vi "DAQ_DC-RMS Current Meas Configure and Measure.vi"(0 "DAQmx Task In":refnum<k21>, 2 "Execution Settings":T2, 5 "Range and Terminal Settings":T7={"Global Settings"={"Min Range (A)"=-0.01, "Max Range (A)"=0.01, "Terminal Configuration"=10083, "Shunt Resistor (Ohm)"=0.001}, "Specific Channel Settings"=[]} {"Specific Channel Settings"."Shunt Resistor (ohms)" format="%.2p"; "Specific Channel Settings"."Terminal Configuration" items=["RSE"=10083, "NRSE"=10078, "Differential"=10106]; "Specific Channel Settings"."Max Range" format="%.2p"; "Specific Channel Settings"."Min Range" format="%.2p"; "Global Settings"."Shunt Resistor (Ohm)" format="%.2p"; "Global Settings"."Terminal Configuration" items=["RSE"=10083, "NRSE"=10078, "Differential"=10106]; "Global Settings"."Max Range (A)" format="%.2p"; "Global Settings"."Min Range (A)" format="%.2p"}, 7 "Timing & Trigger Settings":T4={"Timing Settings"={"Sample Clock Source"="OnboardClock", "Sample Rate (Hz)"=10000.0, "Number of Samples"=1000, "Sample Timing Engine"=enum."Auto"}, "Trigger Settings"={"Trigger Type"=enum."No Trigger", "Digital Start Trigger Source"="", "Digital Start Trigger Edge"=10280}} {"Trigger Settings"."Digital Start Trigger Edge" items=["Rising"=10280, "Falling"=10171]; "Timing Settings"."Sample Rate (Hz)" format="%.2p"}, 11 "error in":errorcluster) -> (4 "DAQmx Task Out":refnum<k21>, 6 "DC and RMS Current Measurements":T1 {"RMS Current (A)" format="%#.2p"; "Average DC Current (A)" format="%#.2p"}, 8 "Current Waveforms":waveform(dbl)[](graph), 10 "Acquisition Time (s)":dbl format="%.2p", 15 "error out":errorcluster)   [LabVIEW 2021, in "DAQ_DC-RMS Current Measurement.lvlib"]
doc: "Configure, initiate and fetch DC-RMS Current measurements from the channels configured."
uses:
  DAQ_DC-RMS Current Measurement.lvlib
  Typedefs/Range and Terminal Settings.ctl
  Typedefs/Specific Channel Settings.ctl
  Typedefs/Timing & Trigger Settings.ctl
  Typedefs/Timing Settings.ctl
  Typedefs/Trigger Settings.ctl
  Typedefs/Execution Settings.ctl
  Common/Typedefs/Execution Options - Measure.ctl
  Typedefs/DC and RMS Current Measurements.ctl
  <vilib>/DAQmx/read.llb/DAQmx Read (Analog 1D Wfm NChan NSamp).vi
  <vilib>/DAQmx/configure/timing.llb/DAQmx Timing (Sample Clock).vi
  <vilib>/DAQmx/configure/trigger.llb/DAQmx Start Trigger (Digital Edge).vi
  <vilib>/DAQmx/miscellaneous.llb/DAQmx Fill In Error Info.vi
  <resource>/objmgr/daqmx.rc
panel:
  # "Inputs"
  # "Outputs"
  # "Min. Range(A)"
  # "Max. Range(A)"
  # "Terminal Configuration"
  # "Shunt\nResistor(Ohm)"
  # "Physical Channel Name"
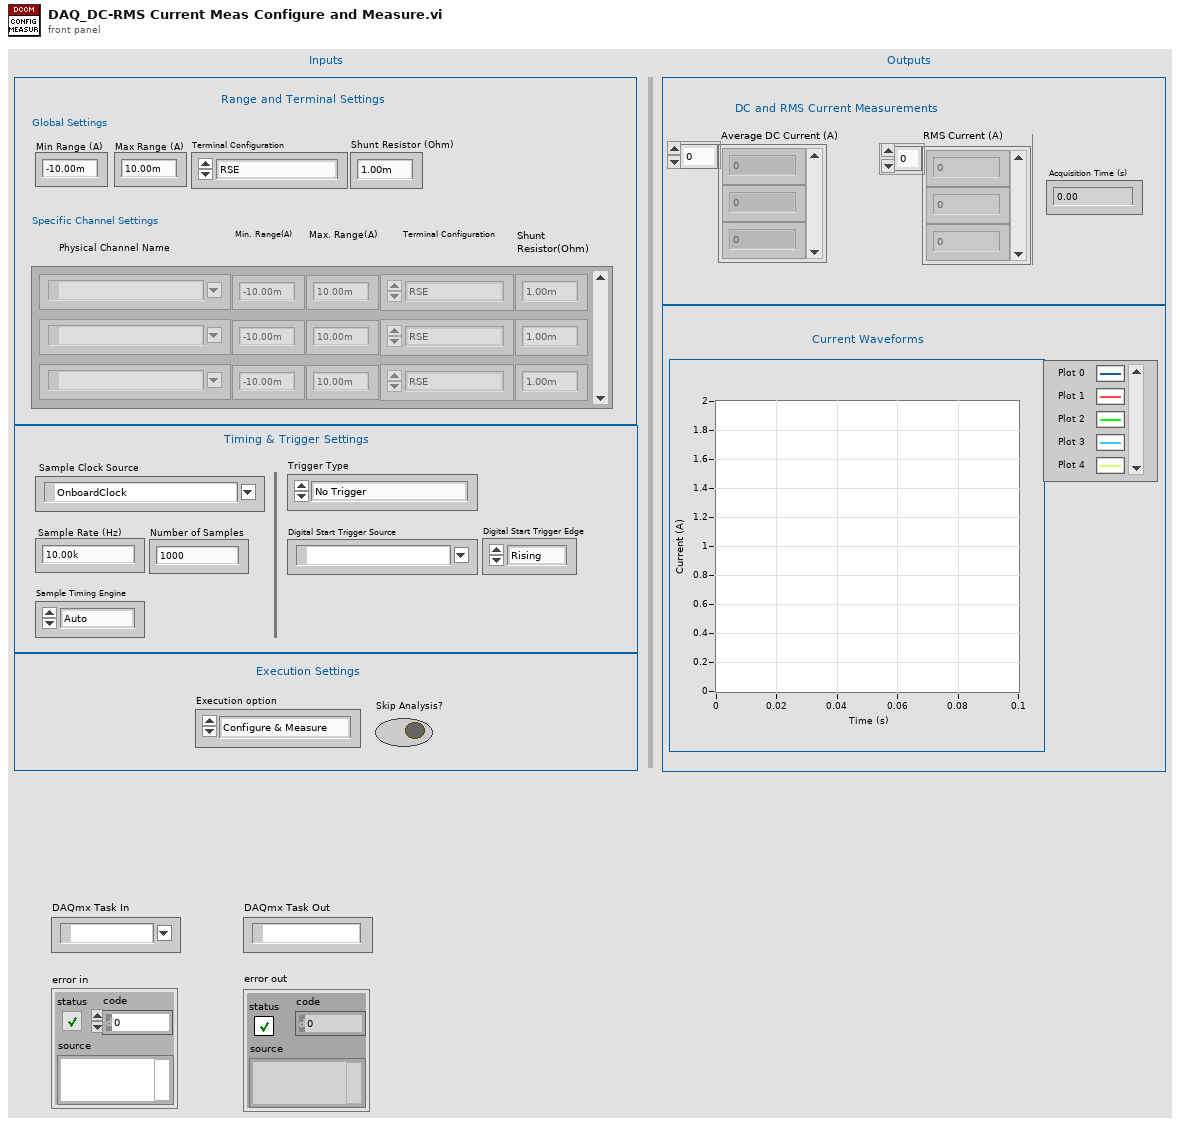
[diagram p1: front panel]
types:
  T1 = typedef "DAQ_DC-RMS Current Measurement.lvlib/DC and RMS Current Measurements.ctl" = cluster{"Average DC Current (A)":dbl[], "RMS Current (A)":dbl[]}
  T2 = typedef "DAQ_DC-RMS Current Measurement.lvlib/Execution Settings.ctl" = cluster{"Execution option":T3, "Skip Analysis?":bool}
  T3 = typedef "Execution Options - Measure.ctl" = enum16{"Configure & Measure", "Configure only", "Measure only"}
  T4 = typedef "DAQ_DC-RMS Current Measurement.lvlib/Timing & Trigger Settings.ctl" = cluster{"Timing Settings":T5, "Trigger Settings":T6}
  T5 = typedef "DAQ_DC-RMS Current Measurement.lvlib/Timing Settings.ctl" = cluster{"Sample Clock Source":tag, "Sample Rate (Hz)":dbl, "Number of Samples":i32, "Sample Timing Engine":enum16{"te0", "te1", "ai", "Auto"}}
  T6 = typedef "DAQ_DC-RMS Current Measurement.lvlib/Trigger Settings.ctl" = cluster{"Trigger Type":enum16{"No Trigger", "Digital Start"}, "Digital Start Trigger Source":tag, "Digital Start Trigger Edge":i32}
  T7 = typedef "DAQ_DC-RMS Current Measurement.lvlib/Range and Terminal Settings.ctl" = cluster{"Global Settings":cluster{"Min Range (A)":dbl, "Max Range (A)":dbl, "Terminal Configuration":i32, "Shunt Resistor (Ohm)":dbl}, "Specific Channel Settings":T8[]}
  T8 = typedef "DAQ_DC-RMS Current Measurement.lvlib/Specific Channel Settings.ctl" = cluster{"Active Channels":tag, "Min Range":dbl, "Max Range":dbl, "Terminal Configuration":i32, "Shunt Resistor (ohms)":dbl}
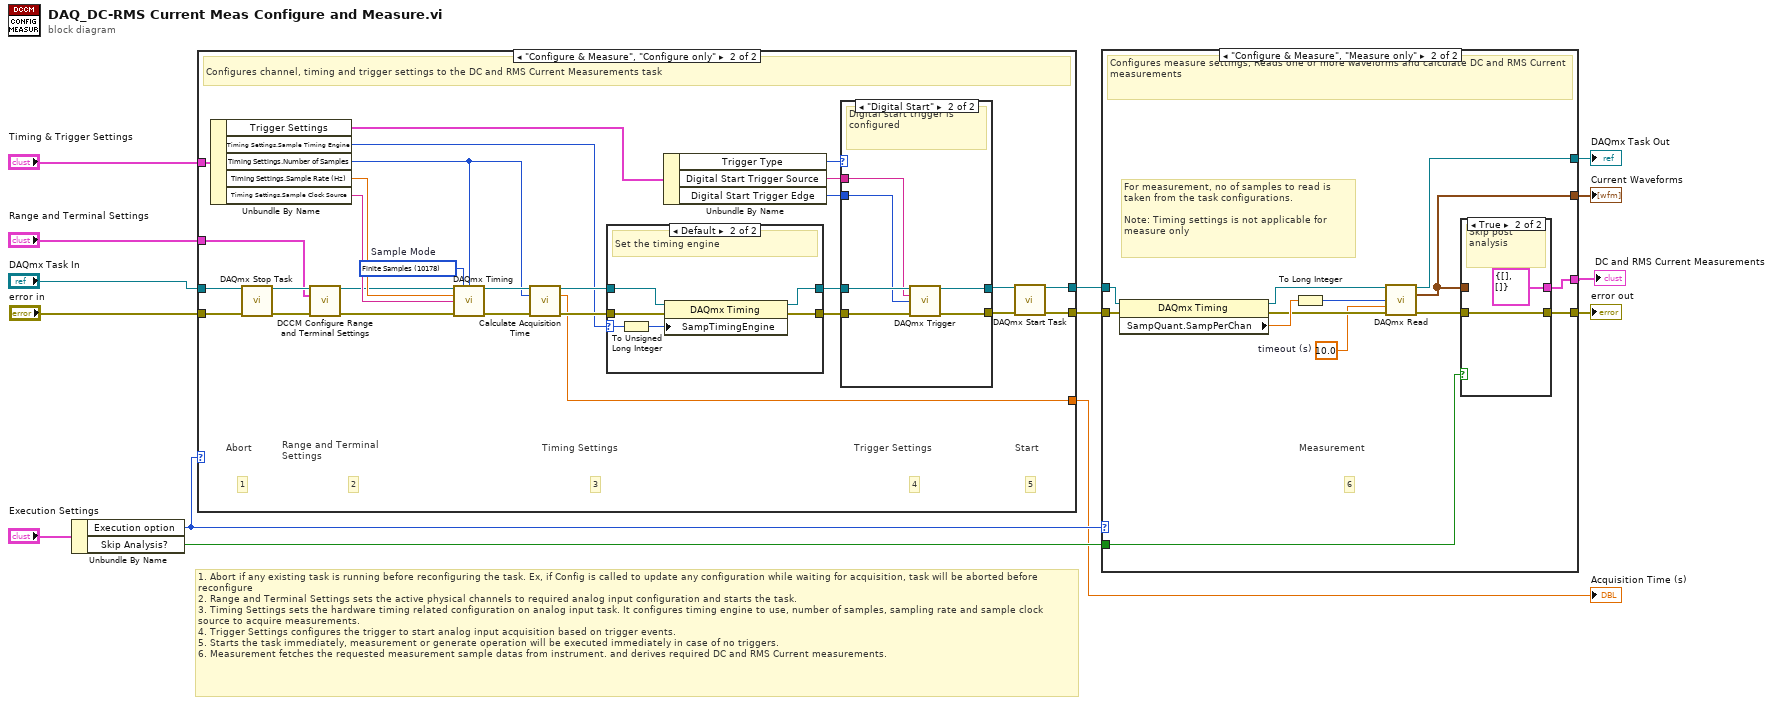
[diagram p0: block diagram]
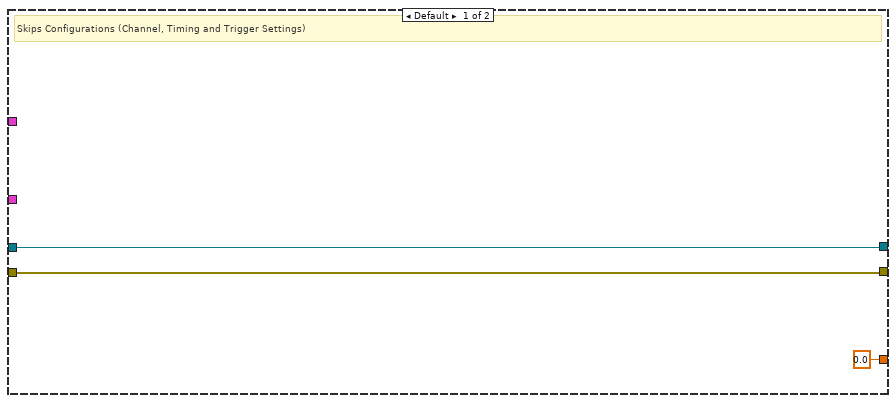
[diagram p2: hidden frame]
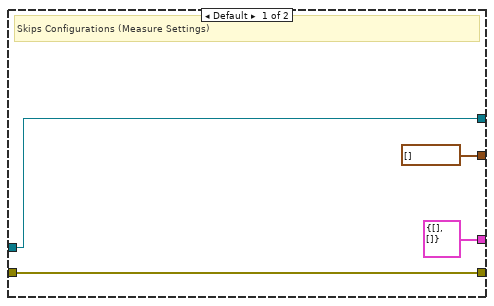
[diagram p5: hidden frame]
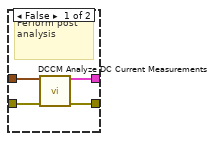
[diagram p6: hidden frame]
diagram:
  # "1. Abort if any existing task is running before reconfiguring the task. Ex, if Config is called to update any configuration while waiting for acquisition, task will be aborted before reconfigure\n2. Range and Terminal Settings sets the active physical channels to required analog input configuration and starts the task.\n3. Timing Settings sets the hardware timing related configuration on analog input task. It configures timing engine to use, number of samples, sampling rate and sample clock source to acquire measurements.\n4. Trigger Settings configures the trigger to start analog input acquisition based on trigger events.\n5. Starts the task immediately, measurement or generate operation will be executed immediately in case of no triggers.\n6. Measurement fetches the requested measurement sample datas from instrument. and derives required DC and RMS Current measurements."
  n1 = Unbundle By Name("Execution Settings") -> ("Execution option"=w4:T3, "Skip Analysis?"=w3:bool)
  n2 = case shown="\"Configure & Measure\", \"Configure only\"" w4 {
    tunnel: "error in" -> [w16 w24]
    tunnel: "DAQmx Task In" -> [w17 w23]
    tunnel: "Range and Terminal Settings" -> [_ w22]
    tunnel: "Timing & Trigger Settings" -> [_ w21]
    tunnel: [w17 w20] -> w6
    tunnel: [w16 w19] -> w7
    tunnel: [0.0 ("Acquisition Time Period (s)") w18] -> w2
    frame Default {
      # "Skips Configurations (Channel, Timing and Trigger Settings)"
    }
    frame "Configure & Measure", "Configure only" {
      w43 = 10178 items=["Finite Samples"=10178, "Continuous Samples"=10123, "Hardware Timed Single Point"=12522]  # Sample Mode
      # "5"
      # "Start"
      # "1"
      # "Abort"
      # "4"
      # "3"
      # "2"
      # "Range and Terminal \nSettings"
      # "Trigger Settings"
      # "Timing Settings"
      # "Configures channel, timing and trigger settings to the DC and RMS Current Measurements task"
      n3 = Unbundle By Name(w21) -> ("Trigger Settings"=w28:T6, "Timing Settings.Sample Timing Engine"=w35:enum16{"te0", "te1", "ai", "Auto"}, "Timing Settings.Number of Samples"=w34:i32, "Timing Settings.Sample Rate (Hz)"=w40:dbl, "Timing Settings.Sample Clock Source"=w41:tag)
      n4 = call <vilib>:"DAQmx Stop Task.vi"("task/channels in"=w23, "error in"=w24) -> ("task out"=w27:refnum<k21>, "error out"=w26:errorcluster)  [unwired: 12 in]
      n5 = call "DCCM Configure Range and Terminal Settings.vi"("DAQmx Task In"=w27, "Range and Terminal Settings"=w22, "error in (no error)"=w26) -> ("DAQmx Task Out"=w29:refnum<k21>, "error out"=w30:errorcluster)  [unwired: 11 in]
      n6 = call-poly <vilib>:"DAQmx Timing.vi"("task/channels in"=w29, "sample mode"=w43, "samples per channel"=w34, "rate"=w40, "source"=w41, "error in"=w30) -> ("task out"=w45:refnum<k21>, "error out"=w44:errorcluster)  [unwired: 8 in]
      n7 = call "Calculate Acquisition Time.vi"("Refnum in"=w45, "Number of Samples"=w34, "error in (no error)"=w44) -> ("Refnum out"=w37:refnum<k21>, "Acquisition Time Period (s)"=w18:dbl, "error out"=w42:errorcluster)  [unwired: 10 in]
      n8 = case shown="Default" w35 {
        selector: w35 -> [_ w49]
        tunnel: w42 -> [w47 w53]
        tunnel: [w47 w52] -> w38
        tunnel: w37 -> [w46 w51]
        tunnel: [w46 w50] -> w36
        frame "Auto" {
          # "Timing engine is auto-selected"
        }
        frame Default {
          # "Set the timing engine"
          n9 = To Unsigned Long Integer(number=w49) -> (unsigned 32bit integer=w48:u32)
          n10 = property class="DAQmx Timing"(reference=w51, error in=w53, "SampTimingEngine"=w48) -> (reference out=w50:refnum<k21>, error out=w52:errorcluster)
        }
      }
      n11 = Unbundle By Name(w28) -> ("Trigger Type"=w31:enum16{"No Trigger", "Digital Start"}, "Digital Start Trigger Source"=w33:tag, "Digital Start Trigger Edge"=w32:i32)
      n12 = case shown="\"Digital Start\"" w31 {
        tunnel: w36 -> [w55 w61]
        tunnel: w38 -> [w54 w60]
        tunnel: [w55 w59] -> w25
        tunnel: [w54 w58] -> w39
        tunnel: w33 -> [_ w57]
        tunnel: w32 -> [_ w56]
        frame Default {
          # "No Trigger settings has been configured"
        }
        frame "Digital Start" {
          # "Digital start trigger is configured"
          n13 = call-poly <vilib>:"DAQmx Trigger.vi"("task/channels in"=w61, "source"=w57, "edge"=w56, "error in"=w60) -> ("task out"=w59:refnum<k21>, "error out"=w58:errorcluster)  [unwired: 10 in]
        }
      }
      n14 = call <vilib>:"DAQmx Start Task.vi"("task/channels in"=w25, "error in"=w39) -> ("task out"=w20:refnum<k21>, "error out"=w19:errorcluster)  [unwired: 12 in]
    }
  }
  "Acquisition Time (s)" <- w2
  n15 = case shown="\"Configure & Measure\", \"Measure only\"" w4 {
    tunnel: [w64 w76] -> w14
    tunnel: [w65 w78] -> w12
    tunnel: [T1 {"Average DC Current (A)"=[], "RMS Current (A)"=[]} ("DC Measurements") w75] -> w1
    tunnel: [waveform(dbl)[] [] ("data") w74] -> w8
    tunnel: w7 -> [w65 w72]
    tunnel: w6 -> [w64 w70]
    tunnel: w3 -> [_ w66]
    frame Default {
      # "Skips Configurations (Measure Settings)"
    }
    frame "Configure & Measure", "Measure only" {
      w67 = 10.0  # timeout (s)
      # "For measurement, no of samples to read is taken from the task configurations.\n\nNote: Timing settings is not applicable for measure only"
      # "6"
      # "Measurement"
      # "Configures measure settings, Reads one or more waveforms and calculate DC and RMS Current measurements"
      n16 = property class="DAQmx Timing"(reference=w70, error in=w72) -> (reference out=w69:refnum<k21>, error out=w71:errorcluster, "SampQuant.SampPerChan"=w73:dbl)
      n17 = To Long Integer(number=w73) -> (32bit integer=w68:i32)
      n18 = call-poly <vilib>:"DAQmx Read.vi"("task/channels in"=w69, "number of samples per channel"=w68, "timeout"=w67, "error in"=w71) -> ("task out"=w76:refnum<k21>, "data"=w74:waveform(dbl)[], "error out"=w77:errorcluster)  [unwired: 9 in]
      n19 = case shown="True" w66 {
        tunnel: [w81 w84] -> w78
        tunnel: w77 -> [w82 w84]
        tunnel: [w79 T1 {"Average DC Current (A)"=[], "RMS Current (A)"=[]} ("DC Measurements")] -> w75
        tunnel: w74 -> [w80 _]
        frame False {
          # "Perform post analysis"
          n20 = call "DCCM Analyze DC Current Measurements.vi"("Current Waveforms"=w80, "error in (no error)"=w82) -> ("DC and RMS Current Measurements"=w79:T1, "error out"=w81:errorcluster)  [unwired: 12 in]
        }
        frame True {
          # "Skip post analysis"
        }
      }
    }
  }
  "error out" <- w12
  "DAQmx Task Out" <- w14
  "Current Waveforms" <- w8
  "DC and RMS Current Measurements" <- w1
